vi "TDMS Select Dialog.vi"(8 "error in (no error)":errorcluster, 10 "Node":string="Controller/Custom Devices", 11 "WorkspaceManager":T1) -> (0 "error out":errorcluster, 1 "Cancelled?":bool, 2 "Channel":string, 3 "WorkspaceManager out":T1)   [LabVIEW 2011]
uses:
  <vilib>/NI Veristand/Execution/Workspace/WorkspaceAPI.ctl
  NationalInstruments.VeriStand.ClientAPI
  <vilib>/regexp/Match Regular Expression.xnode
  <vilib>/NI Veristand/Execution/Workspace/NI_VS Workspace ExecutionAPI.lvlib
panel:
  in  "OK":bool
  in  "TDMS Custom Device":i32(ring)
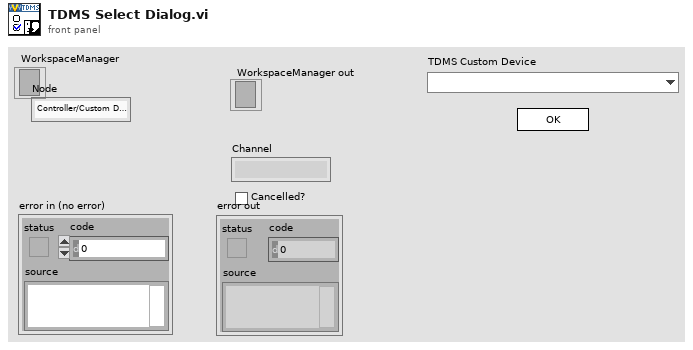
[diagram p1: front panel]
types:
  T1 = typedef "NI_VS Workspace ExecutionAPI.lvlib/WorkspaceAPI.ctl" = refnum<k24>
  T2 = typedef "NI_VS Workspace ExecutionAPI.lvlib/NodeInfo.ctl" = cluster{"Name":string, "FullPath":string, "Type":string, "IsChannel":bool, "Channel":cluster{"Unit":string, "Readable":bool, "Writable":bool, "Faultable":bool, "Scalable":bool, "RowDim":u32, "ColumnDim":u32}}
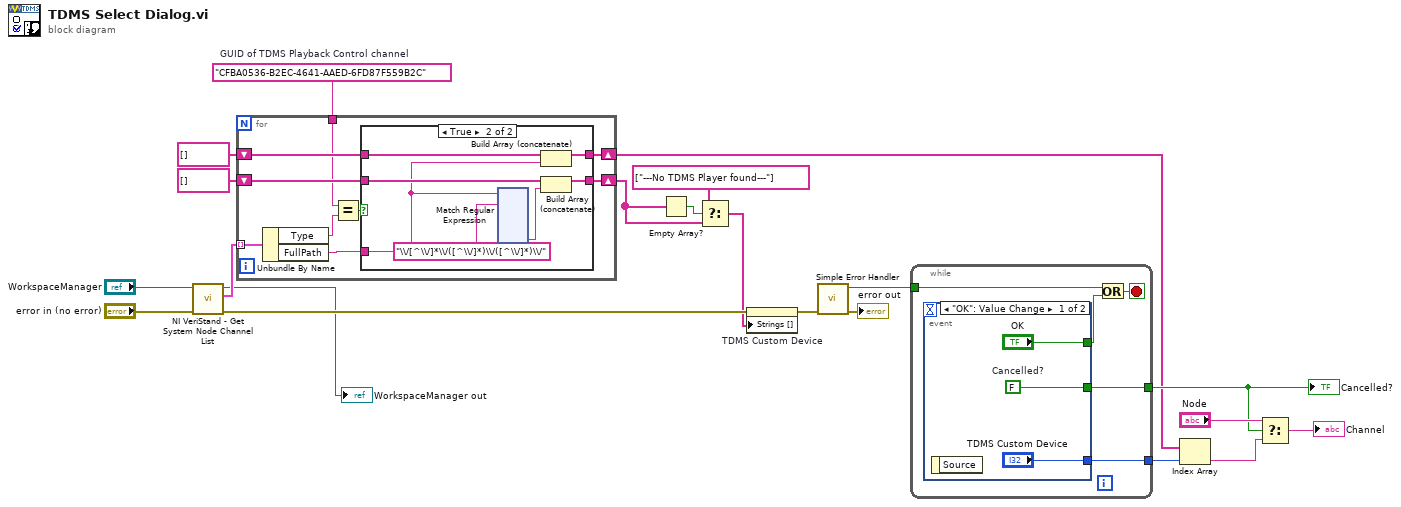
[diagram p0: block diagram]
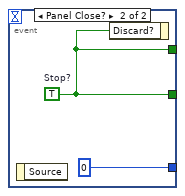
[diagram p3: hidden frame]
diagram:
  w1 = "CFBA0536-B2EC-4641-AAED-6FD87F559B2C"  # GUID of TDMS Playback Control channel
  n1 = call <vilib>:"NI VeriStand - Get System Node Channel List.vi"("error in (no error)"="error in (no error)", "WorkspaceManager in"="WorkspaceManager") -> ("error out"=w17:errorcluster, "Channels"=w21:T2[], "WorkspaceManager out"=→"WorkspaceManager out":T1)  [unwired: 7 in]
  n2 = for {
    tunnel: w21 -> [w30] mode=indexing
    shift-right: [w25] -> w6
    shift-left: string[] [] -> [w26]
    shift-right: [w24] -> w4
    shift-left: string[] [] -> [w23]
    tunnel: w1 -> [w22]
    n3 = Unbundle By Name(w30) -> ("Type"=w29:string, "FullPath"=w27:string)
    n4 = Equal?(x=w22, y=w29) -> (x = y?=w28:bool)
    n5 = case shown="True" w28 {
      tunnel: w27 -> [_ w34]
      tunnel: w26 -> [w32 w39]
      tunnel: [w32 w38] -> w25
      tunnel: [w31 w37] -> w24
      tunnel: w23 -> [w31 w36]
      frame False {
      }
      frame True {
        n6 = xnode "Match Regular Expression"("input string"=w34, "regular expression"="\\/[^\\/]*\\/([^\\/]*)\\/([^\\/]*)\\/") -> ("submatch 2"=w33:string)  [unwired: 2 in, 8 out]
        n7 = Build Array (concatenate)(w39, w34) -> (w38:string[])
        n8 = Build Array (concatenate)(w36, w33) -> (w37:string[])
      }
    }
  }
  n9 = Empty Array?(array=w4) -> (empty?=w5:bool)
  n10 = Select(t=string[] ["---No TDMS Player found---"], s=w5, f=w4) -> (s? t:f=w2:string[])
  n11 = property on="TDMS Custom Device" class="Ring (strict)"(error in=w17, "Strings []"=w2) -> (error out=w16:errorcluster)  [unwired: 1 in, 1 out]
  n12 = call <vilib>:"Simple Error Handler.vi"("error in (no error)"=w16) -> ("error?"=w15:bool, "error out"=→"error out":errorcluster)  [unwired: 1 in, 6 out]
  n13 = while {
    tunnel: [w158] -> w8
    tunnel: [w157] -> w12
    tunnel: w15 -> [w154]
    stop <- w156 stop-if-true
    n14 = event shown="[0] \"OK\": Value Change" {
      selector: _ -> [_ _]
      dyn-events: _ -> [_ _]
      timeout: _ -> [_ _]
      tunnel: ["OK" w163] -> w155
      tunnel: [w161 w163] -> w158
      tunnel: ["TDMS Custom Device" 0 ("TDMS Custom Device")] -> w157
      event "OK": Value Change {
        w161 = FALSE  # Cancelled?
        n15 = event-data() -> ()  [unwired: 2 out]
      }
      event Panel Close? {
        w163 = TRUE  # Stop?
        n16 = event-data() -> ()  [unwired: 2 out]
        n17 = event-data("Discard?"=w163) -> ()  [unwired: 1 in, 1 out]
      }
    }
    n18 = Or(x=w154, y=w155) -> (x .or. y?=w156:bool)
  }
  "Cancelled?" <- w8
  n19 = Index Array(array=w6, index=w12) -> (element=w10:string)
  n20 = Select(t="Node", s=w8, f=w10) -> (s? t:f=→"Channel":string)
